vi "PH_4_Pos_Selector.set i Attr and start DIM Services.vi"(0 "i ref in":refnum<vi>, 5 "error in (no error)":errorcluster) -> (14 "i ref out":refnum<vi>, 15 "Wanted start position":T1 items=["unknown", "Position I", "Position II", "Position III", "Position IV", "moving"], 16 "i Attr":T2 {"Current Position" items=["unknown", "Position I", "Position II", "Position III", "Position IV", "moving"]}, 19 "error out":errorcluster)   [LabVIEW 2014, in "PH_4_Pos_Selector.lvlib"]
doc: "This VI reads the DB special 0 and 1 DB entries which are the axis names and writes them to own attributes. Depending on this, several GUI elements are set."
uses:
  PH_4_Pos_Selector.lvlib
  PH_4_Pos_Selector.i attribute.ctl
  PH_4_Pos_Selector.Position Selector.ctl
  PH_4_Pos_Selector.Position.ctl
  PH_Basics/PH_Common/PH_Common.lvlib
  CS_Core/CSSystem/CSSystemLib/CSSystemLib.lvlib
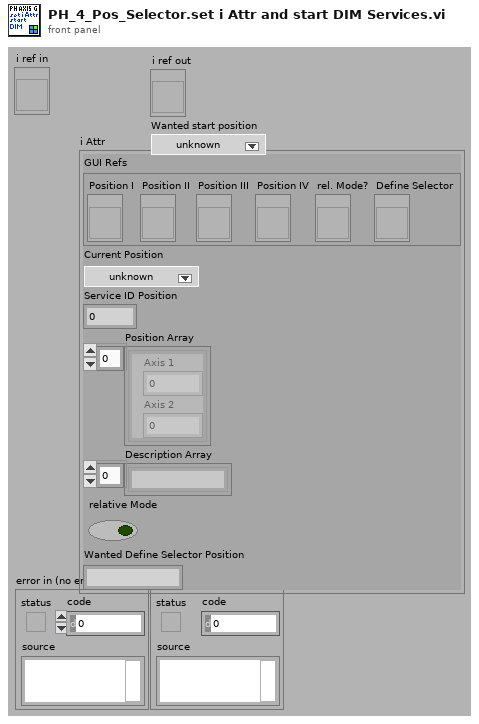
[diagram p1: front panel]
types:
  T1 = typedef "PH_4_Pos_Selector.lvlib/PH_4_Pos_Selector.Position Selector.ctl" = u16
  T2 = typedef "PH_4_Pos_Selector.lvlib/PH_4_Pos_Selector.i attribute.ctl" = cluster{"GUI Refs":cluster{"Position I":refnum<vi>, "Position II":refnum<vi>, "Position III":refnum<vi>, "Position IV":refnum<vi>, "rel. Mode?":refnum<vi>, "Define Selector":refnum<vi>}, "Current Position":T1, "Service ID Position":i32, "Position Array":T3[], "Description Array":string[], "relative Mode":bool, "Wanted Define Selector Position":string}
  T3 = typedef "PH_4_Pos_Selector.lvlib/PH_4_Pos_Selector.Position.ctl" = cluster{"Axis 1":dbl, "Axis 2":dbl}
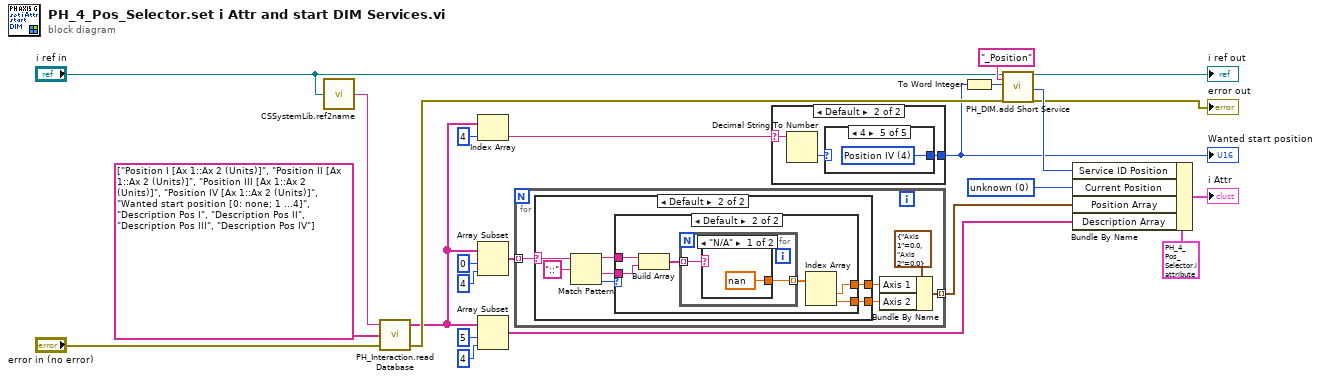
[diagram p0: block diagram]
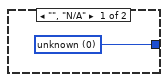
[diagram p2: hidden frame]
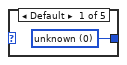
[diagram p3: hidden frame]
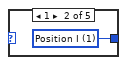
[diagram p4: hidden frame]
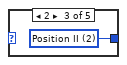
[diagram p5: hidden frame]
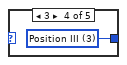
[diagram p6: hidden frame]
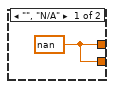
[diagram p7: hidden frame]
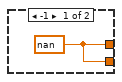
[diagram p8: hidden frame]
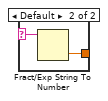
[diagram p9: hidden frame]
diagram:
  w17 = T1 0 items=["unknown", "Position I", "Position II", "Position III", "Position IV"] ("Selector")
  n1 = call "CSSystemLib.ref2name.vi"("obj refnum"="i ref in") -> ("name"=w9:string)
  n2 = call "PH_Interaction.read Database.vi"("error in (no error)"="error in (no error)", "Strings to search for"=string[] ["Position I [Ax 1::Ax 2 (Units)]", "Position II [Ax 1::Ax 2 (Units)]", "Position III [Ax 1::Ax 2 (Units)]", "Position IV [Ax 1::Ax 2 (Units)]", "Wanted start position [0: none; 1 ...4]", "Description Pos I", "Description Pos II", "Description Pos III", "Description Pos IV"] ("Strings to search for in"), "DB Entry to read"=w9) -> ("error out"=w11:errorcluster, "Values"=w4:string[])  [unwired: 1 in]
  n3 = Index Array(array=w4, index=4) -> (element=w20:string)
  n4 = Array Subset(array=w4, index=0, length=4) -> (w22:string[])
  n5 = Array Subset(array=w4, index=5, length=4) -> (w2:string[])
  n6 = for {
    tunnel: w22 -> [w27] mode=indexing
    tunnel: [w26] -> w3 mode=indexing
    n7 = case shown="Default" w27 {
      selector: w27 -> [_ w31]
      tunnel: [w30 w33] -> w29
      tunnel: [w30 w32] -> w28
      frame "", "N/A" {
        w30 = nan
      }
      frame Default {
        n8 = Match Pattern(string=w31, regular expression="::") -> (before substring=w36:string, after substring=w35:string, offset past match=w34:i32)  [unwired: 1 in, 1 out]
        n9 = case shown="Default" w34 {
          tunnel: w36 -> [_ w44]
          tunnel: w35 -> [_ w43]
          tunnel: [w38 w40] -> w33
          tunnel: [w38 w39] -> w32
          frame -1 {
            w38 = nan
          }
          frame Default {
            n10 = Build Array(w44, w43) -> (w42:string[])
            n11 = for {
              tunnel: w42 -> [w45] mode=indexing
              tunnel: [w46] -> w41 mode=indexing
              n12 = case shown="\"N/A\"" w45 {
                selector: w45 -> [_ w48]
                tunnel: [nan w49] -> w46
                frame "N/A" {
                }
                frame Default {
                  n13 = Fract/Exp String To Number(string=w48) -> (number=w49:dbl)  [unwired: 3 in, 1 out]
                }
              }
            }
            n14 = Index Array(array=w41) -> (element #1=w40:dbl, element #2=w39:dbl)  [unwired: 2 in]
          }
        }
      }
    }
    n15 = Bundle By Name(cluster=T3 {"Axis 1"=0.0, "Axis 2"=0.0} ("Position"), "Axis 1"=w29, "Axis 2"=w28) -> (w26:T3)
  }
  n16 = case shown="Default" w20 {
    selector: w20 -> [_ w53]
    tunnel: [w50 w51] -> w1
    frame "", "N/A" {
      w50 = T1 0 items=["unknown", "Position I", "Position II", "Position III", "Position IV"] ("Wanted Position")
    }
    frame Default {
      n17 = Decimal String To Number(string=w53) -> (number=w52:i32)  [unwired: 2 in, 1 out]
      n18 = case shown="4" w52 {
        tunnel: [w54 w55 w56 w57 w58] -> w51
        frame Default {
          w54 = T1 0 items=["unknown", "Position I", "Position II", "Position III", "Position IV"] ("Wanted Position")
        }
        frame 1 {
          w55 = T1 1 items=["unknown", "Position I", "Position II", "Position III", "Position IV"] ("Wanted Position")
        }
        frame 2 {
          w56 = T1 2 items=["unknown", "Position I", "Position II", "Position III", "Position IV"] ("Wanted Position")
        }
        frame 3 {
          w57 = T1 3 items=["unknown", "Position I", "Position II", "Position III", "Position IV"] ("Wanted Position")
        }
        frame 4 {
          w58 = T1 4 items=["unknown", "Position I", "Position II", "Position III", "Position IV"] ("Wanted Position")
        }
      }
    }
  }
  "Wanted start position" <- w1
  n19 = To Word Integer(number=w1) -> (16bit integer=w18:i16)
  n20 = call "PH_DIM.add Short Service.vi"("i ref in"="i ref in", "Service Name"="_Position", "Number"=w18, "error in (no error)"=w11) -> ("i ref out"=→"i ref out":refnum<vi>, "Service ID"=w19:i32, "error out"=→"error out":errorcluster)  [unwired: 13 in]
  n21 = Bundle By Name(cluster=T2 {"GUI Refs"={"Position I"=refnum, "Position II"=refnum, "Position III"=refnum, "Position IV"=refnum, "rel. Mode?"=refnum, "Define Selector"=refnum}, "Current Position"=0, "Service ID Position"=0, "Position Array"=[], "Description Array"=[], "relative Mode"=FALSE, "Wanted Define Selector Position"=""} ("CLASS.i attribute"), "Service ID Position"=w19, "Current Position"=w17, "Position Array"=w3, "Description Array"=w2) -> (→"i Attr":T2)
